vi "Tray_ArrAndData.vi"() -> ()   [LabVIEW 2019]
uses:
  NozzelUse/Ctrl/Nozzel_Tray_main.ctl
panel:
  out "Arr_TrayD_ 2":cluster{"X":sgl, "Y":sgl}[][](array[cluster])
  out "Arr_TrayC_ 2":cluster{"X":sgl, "Y":sgl}[][](array[cluster])
  out "Arr_TrayB_ 2":cluster{"X":sgl, "Y":sgl}[][](array[cluster])
  out "Arr_TrayA_ 2":cluster{"X":sgl, "Y":sgl}[][](array[cluster])
  out "IngornePointQue":refnum<queue>
  out "Arr_TrayD_":cluster{"X":sgl, "Y":sgl}[][](array[cluster])
  out "Arr_TrayC_":cluster{"X":sgl, "Y":sgl}[][](array[cluster])
  out "Arr_TrayB_":cluster{"X":sgl, "Y":sgl}[][](array[cluster])
  out "Arr_TrayA_":cluster{"X":sgl, "Y":sgl}[][](array[cluster])
  in  "Stop Ref":refnum<vi>
  in  "IgPanelInsert":bool
  out "mid_NG2":bool[][](array[boolean])
  out "mid_Pass":bool[][](array[boolean])
  out "mid_NG1":bool[][](array[boolean])
  out "mid_Dut":bool[][](array[boolean])
  in  "InputData":string[](array[string])
  in  "PASS From SHB":string[](array[string])
  in  "NGRTrayFromSHB":string[](array[string])
  in  "NGLTrayFromSHB":string[](array[string])
  out "XY_ATray_N2":cluster{"Y1":i32, "Y2":i32} caption="DutTrayN2"
  out "Arr_TrayA_3D_N2":cluster{"X":sgl, "Y":sgl, "Z":sgl}[][](array[cluster])
  out "Arr_TrayD_3D":cluster{"X":sgl, "Y":sgl, "Z":sgl}[][](array[cluster])
  out "Arr_TrayC_3D":cluster{"X":sgl, "Y":sgl, "Z":sgl}[][](array[cluster])
  out "Arr_TrayB3D":cluster{"X":sgl, "Y":sgl, "Z":sgl}[][](array[cluster])
  out "Arr_TrayA_3D_N1":cluster{"X":sgl, "Y":sgl, "Z":sgl}[][](array[cluster])
  in  "TrayRef":refnum<vi>[](array[refnum])
  out "DTray":T1={"XY_DTray"={"X"=0, "Y"=0}, "Initial color"=13816530, "FinalColor"=16711680}
  out "CTray":T2={"XY_CTray"={"X"=0, "Y"=0}, "Initial color"=13816530, "FinalColor"=16711680}
  out "BTray":T3={"XY_BTray"={"X"=0, "Y"=0}, "Initial color"=13816530, "FinalColor"=6618880}
  out "ATray":T4={"XY_ATray"={"X"=0, "Y"=0}, "Initial color"=16860, "FinalColor"=13816530}
  out "Arr_DTray":bool[][](array[boolean]) caption="NGTray Left"
  out "Arr_BTray":bool[][](array[boolean]) caption="PassTray"
  out "Arr_CTray":bool[][](array[boolean]) caption="NGTray Right"
  out "Arr_ATray":bool[][](array[boolean]) caption="DutTray"
  # "手臂端 右一 左二\n              右A  左B\n              右C 左D"
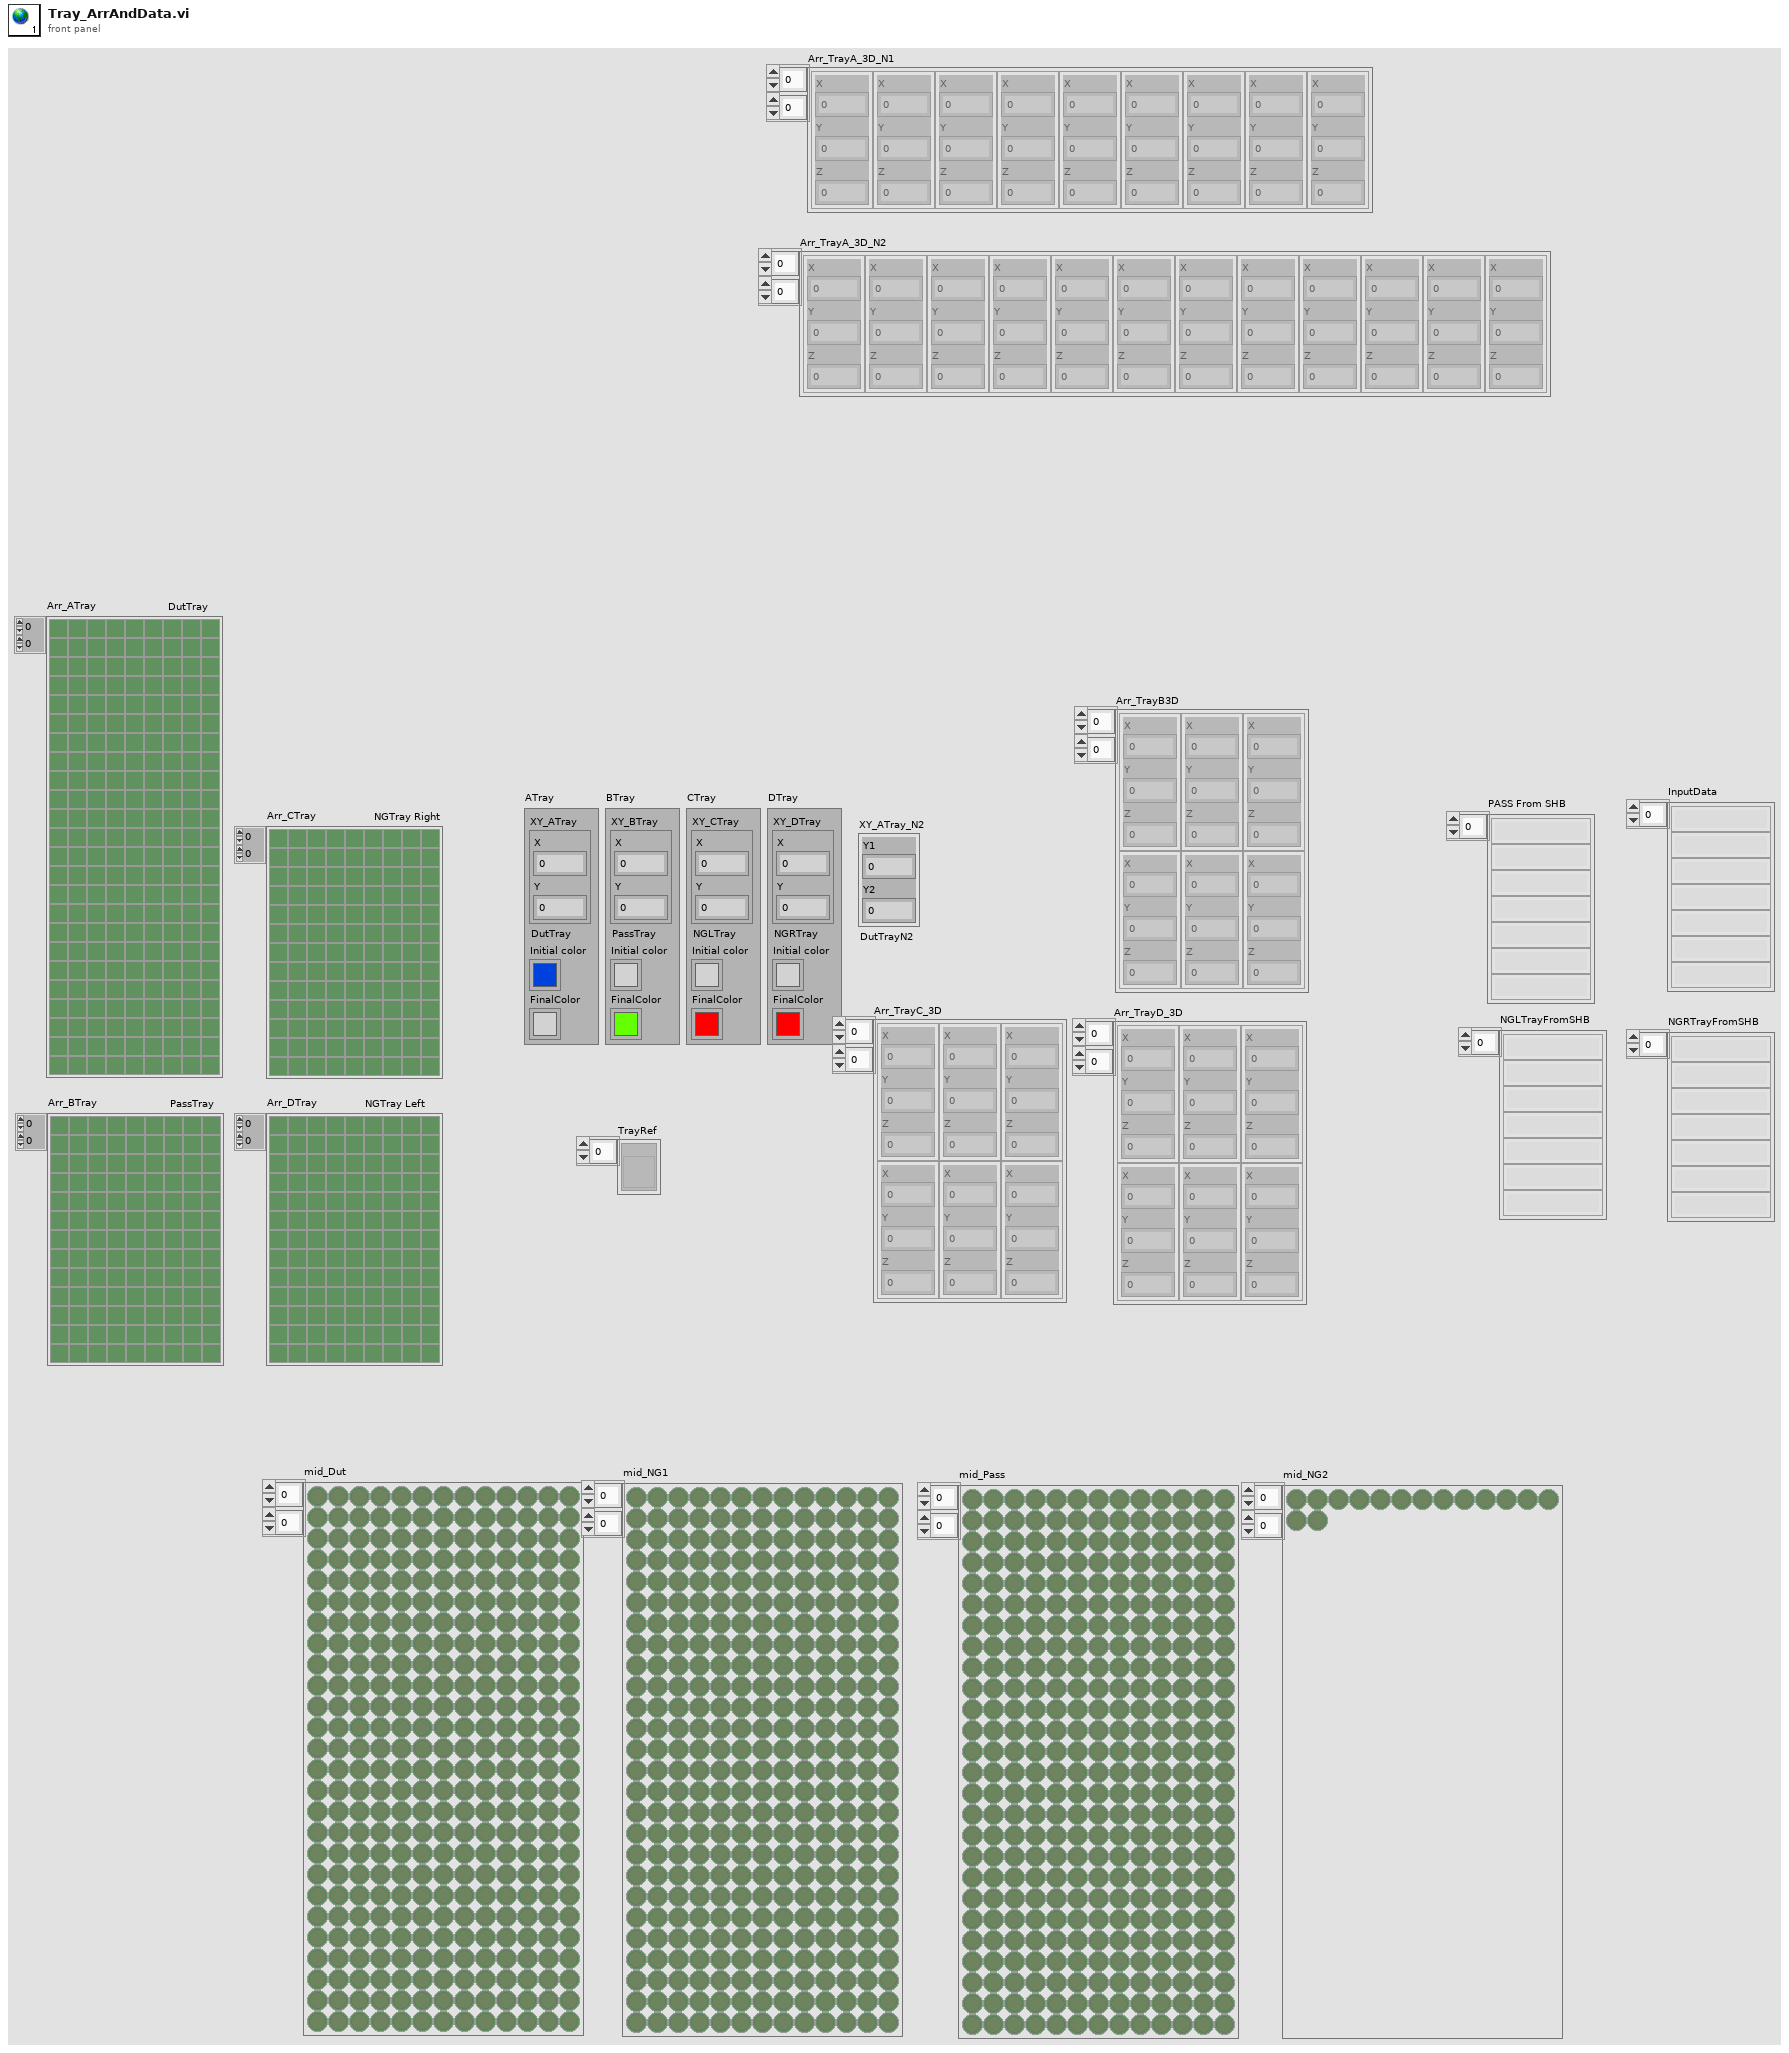
[diagram p1: front panel]
types:
  T1 = cluster{"XY_DTray":cluster{"X":i32, "Y":i32}, "Initial color":u32, "FinalColor":u32}
  T2 = cluster{"XY_CTray":cluster{"X":i32, "Y":i32}, "Initial color":u32, "FinalColor":u32}
  T3 = cluster{"XY_BTray":cluster{"X":i32, "Y":i32}, "Initial color":u32, "FinalColor":u32}
  T4 = cluster{"XY_ATray":cluster{"X":i32, "Y":i32}, "Initial color":u32, "FinalColor":u32}
diagram:
